vi "Post uninstall.vi"(11 "Arguments":string[](array[string])) -> (2 "Output error":string, 3 "Exit code":i32)   [LabVIEW 2021]
uses:
  <vilib>/zip/NI_Unzip.lvlib
  <vilib>/Utility/config.llb/NI_LVConfig.lvlib
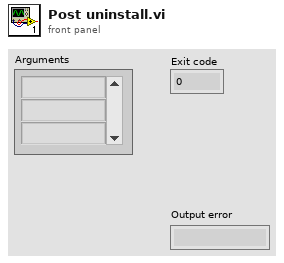
[diagram p1: front panel]
types:
  T1 = typedef "NI_LVConfig.lvlib/Config Data RefNum.ctl" = refnum<k1>
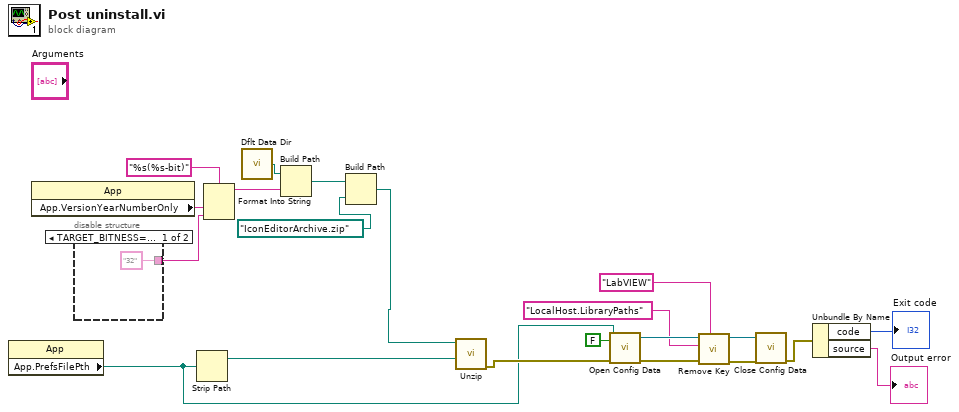
[diagram p0: block diagram]
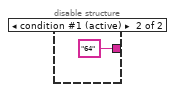
[diagram p2: hidden frame]
diagram:
  n1 = property class="App"() -> ("App.PrefsFilePth"=w4:path)  [unwired: 2 in, 2 out]
  n2 = property class="App"() -> ("App.VersionYearNumberOnly"=w14:string)  [unwired: 2 in, 2 out]
  n3 = disable-structure shown="TARGET_BITNESS==32" {
    disable-tunnel: ["32" "64"] -> w15
    frame condition #0 {
    }
    frame condition #1 (active) {
    }
  }
  n4 = Strip Path(path=w4) -> (stripped path=w6:path)  [unwired: 1 out]
  n5 = Format Into String(format string="%s(%s-bit)", w14, w15) -> (resulting string=w16:string)  [unwired: 2 in, 1 out]
  n6 = call <vilib>:"Dflt Data Dir.vi"() -> ("App:Default Data Directory"=w20:path)
  n7 = Build Path(base path=w20, name or relative path=w16) -> (appended path=w19:path)
  n8 = Build Path(base path=w19, name or relative path=path "IconEditorArchive.zip") -> (appended path=w17:path)
  n9 = call <vilib>:"Unzip.vi"("Target directory (same as Zip file if empty)"=w6, "Zip file"=w17) -> ("error out"=w5:errorcluster)  [unwired: 7 in, 2 out]
  n10 = call <vilib>:"Open Config Data.vi"("error in (no error)"=w5, "create file if necessary (T)"=FALSE, "configuration file path"=w4) -> ("error out"=w13:errorcluster, "refnum"=w12:T1)  [unwired: 6 in, 1 out]
  n11 = call <vilib>:"Remove Key.vi"("section"="LabVIEW", "error in (no error)"=w13, "key"="LocalHost.LibraryPaths", "refnum"=w12) -> ("error out"=w9:errorcluster, "refnum out"=w8:T1)  [unwired: 5 in, 1 out]
  n12 = call <vilib>:"Close Config Data.vi"("error in (no error)"=w9, "refnum"=w8) -> ("error out"=w3:errorcluster)  [unwired: 8 in, 1 out]
  n13 = Unbundle By Name(w3) -> ("code"=→"Exit code":i32, "source"=→"Output error":string)
